vi "Division.vi"() -> ()   [LabVIEW 2013]
panel:
  out "Result":dbl
  in  "Num 2":dbl
  in  "Num 1":dbl
  # "Click          to run"
  # "÷"
  # "="
  # "Division"
  # "The goal of this exercise is simple. Make a calculator that does division. The challenge is that you cannot use the built in divide (or multiply) functions from the mathematics pallete. Only addition and subtraction.\nFurthermore, you must calculate the quotient to four decimal places.\nI would suggest using strings to keep tract of the decimal point. But if you are creative enough to come up with your own method of doing this, that's even better."
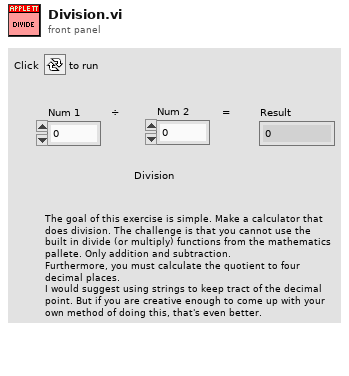
[diagram p1: front panel]
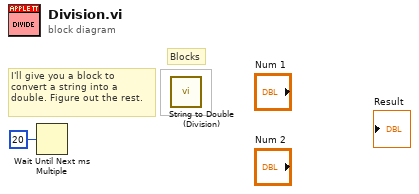
[diagram p0: block diagram]
diagram:
  # "I'll give you a block to convert a string into a double. Figure out the rest."
  # "Blocks"
  n1 = Wait Until Next ms Multiple(millisecond multiple=u32 20) -> ()  [unwired: 1 out]
  n2 = call "String to Double (Division).vi"() -> ()  [unwired: 1 in, 1 out]
